vi "F Dwf Analog IO Channel Node Status Info.vi"(0 "hdwf":i32, 1 "pmax":dbl, 5 "idxChannel":i32, 7 "idxNode":i32, 9 "pmin":dbl, 11 "error in (no error)":errorcluster, 12 "pnSteps":i32) -> (3 "pmax out":dbl, 4 "function return":i32, 10 "pmin out":dbl, 14 "pnSteps out":i32, 15 "error out":errorcluster)   [LabVIEW 2019, in "Olasdwf.lvlib"]
doc: "DWFAPI int FDwfAnalogIOChannelNodeStatusInfo(HDWF hdwf, int idxChannel, int idxNode, double *pmin, double *pmax, int *pnSteps);"
uses:
  Olasdwf.lvlib
  Windows/System32/dwf.dll
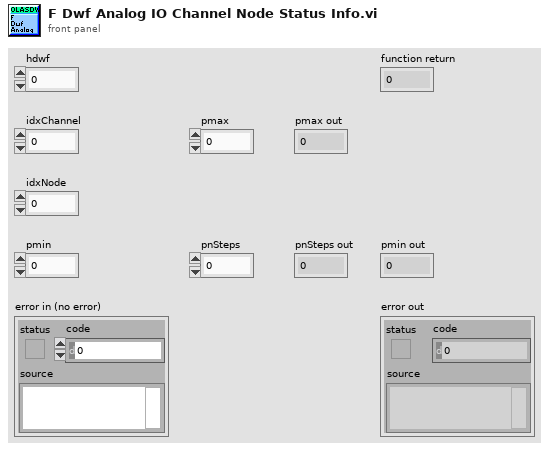
[diagram p1: front panel]
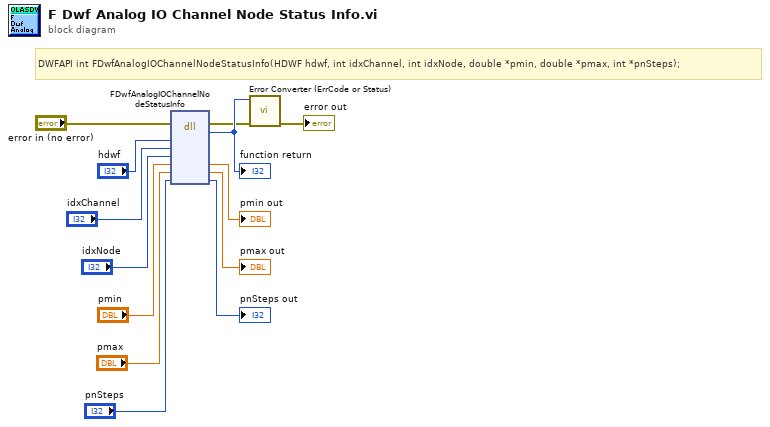
[diagram p0: block diagram]
diagram:
  # "DWFAPI int FDwfAnalogIOChannelNodeStatusInfo(HDWF hdwf, int idxChannel, int idxNode, double *pmin, double *pmax, int *pnSteps);"
  n1 = dll-call lib="C:/Windows/System32/dwf.*" fn="FDwfAnalogIOChannelNodeStatusInfo"(error in="error in (no error)", "hdwf"="hdwf", "idxChannel"="idxChannel", "idxNode"="idxNode", "pmin"="pmin", "pmax"="pmax", "pnSteps"="pnSteps") -> (error out=w2:errorcluster, w13:i32, "pmin"=→"pmin out":dbl, "pmax"=→"pmax out":dbl, "pnSteps"=→"pnSteps out":i32)  [unwired: 5 in, 1 out]
  "function return" <- w13
  n2 = call "Error Converter (ErrCode or Status).vi"("error in (no error)"=w2, "error code"=w13) -> ("error out"=→"error out":errorcluster)  [unwired: 9 in]
